vi "Preview State.vi"(8 "error in (no error)":errorcluster, 11 "He Line in":refnum<class "He Line.lvclass">) -> (0 "error out":errorcluster, 2 "Is Open?":bool, 3 "He Line out":refnum<class "He Line.lvclass">)   [LabVIEW 2015, in "cRIO-Carbondioxide.lvlib" / "CO2-Actor.lvlib" / "He Line.lvclass"]
uses:
  He Line.lvclass
  Valve/Valve.lvclass
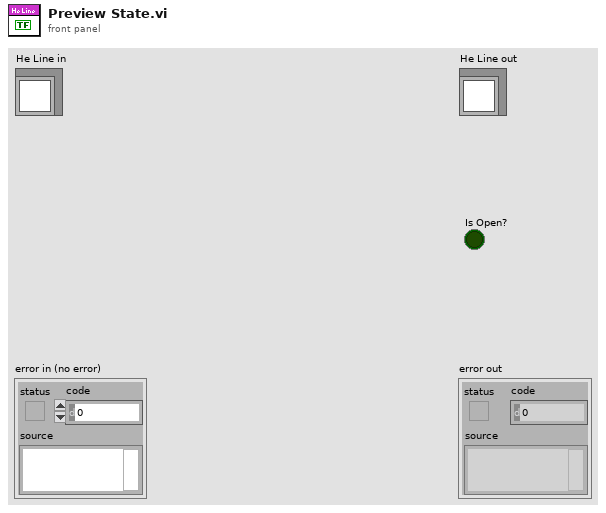
[diagram p1: front panel]
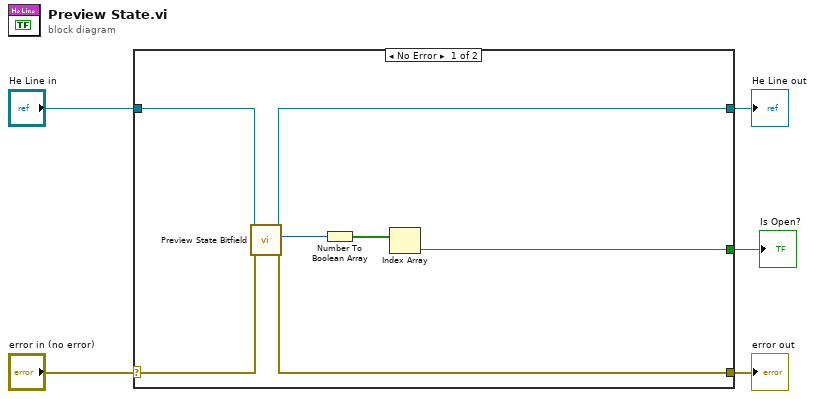
[diagram p0: block diagram]
diagram:
  n1 = case shown="No Error" "error in (no error)" {
    selector: "error in (no error)" -> [w10 w14]
    tunnel: [w9 w14] -> w4
    tunnel: [w11 w13] -> w2
    tunnel: "He Line in" -> [w12 w13]
    tunnel: [w6 _] -> w1
    frame No Error {
      n2 = call "Preview State Bitfield.vi"("error in (no error)"=w10, "Valve in"=w12) -> ("error out"=w9:errorcluster, "State Bitfield"=w8:u16, "Valve out"=w11:refnum<class "He Line.lvclass">)  [unwired: 7 in]
      n3 = Number To Boolean Array(number=w8) -> (Boolean array=w7:bool[])
      n4 = Index Array(array=w7) -> (element=w6:bool)  [unwired: 1 in]
    }
    frame Error {
    }
  }
  "error out" <- w4
  "He Line out" <- w2
  "Is Open?" <- w1
